vi "EXECUTE SWERVE DRIVE.vi"(0 "Swerve refs":cluster{"Driver":T1, "Steer":T1, "Encoder":T6}[](array[cluster]), 5 "HEADING":dbl, 7 "DRIVE MAX SPEED":dbl=0.7, 9 "STEER MAX speed":dbl=0.7) -> (4 "VELOCITIES":dbl[](array[numeric]), 6 "STEERING\nANGLES (deg)":dbl[](array[numeric]))   [LabVIEW 2023]
uses:
  <vilib>/Rock Robotics/WPI/MotorControl/WPI_MotorControlDeviceRef.ctl
  <vilib>/Rock Robotics/WPI/MotorControl/WPI_MotorControlType.ctl
  <vilib>/Rock Robotics/SystemInterfaces/DIO/FPGA_DIOPWMChannel.ctl
  <vilib>/Rock Robotics/WPI/PWM/WPI_PWMDeadband.ctl
  <vilib>/Rock Robotics/SystemInterfaces/DIO/FPGA_DIOChannel.ctl
  <vilib>/Rock Robotics/WPI/ThirdParty/Phoenix-LabVIEW/CANCoder/Controls/CTRE_Phoenix_CANcoder_DeviceRef.ctl
  <vilib>/Rock Robotics/WPI/ThirdParty/REV Robotics/REVLib/Typedef/Spark MAX Control Type.ctl
  Global odometry.vi
  Global INIT.vi
panel:
  out "error out":errorcluster
  in  "error in (no error)":errorcluster
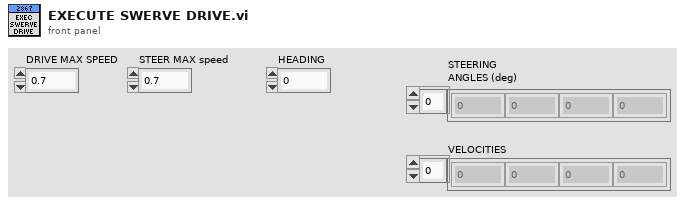
[diagram p1: front panel]
types:
  T1 = typedef "WPI_MotorControlDeviceRef.ctl" = cluster{"DeviceStatus":errorcluster, "Type":T2, "PWM":cluster{"PWM Channel":T3, "DeadBand":T4}, "CAN":cluster{"Device Number":u8, "SetOutput VI Ref":variant, "GetOutput VI Ref":variant, "Enable VI Ref":variant, "Disable VI Ref":variant, "Data":variant}, "Invert":bool, "DIO PWM":cluster{"PWM \"Enable\" Channel":T3, "DIOChannel":T5, "PWM Rate":dbl}}
  T2 = typedef "WPI_MotorControlType.ctl" = enum16{"PWM", "CAN", "DIO PWM"}
  T3 = typedef "FPGA_DIOPWMChannel.ctl" = enum8{"PWM 0", "PWM 1", "PWM 2", "PWM 3", "PWM 4", "PWM 5", "PWM 6", "PWM 7", "PWM 8", "PWM 9", "PWM MXP 0", "PWM MXP 1", "PWM MXP 2", "PWM MXP 3", "PWM MXP 4", "PWM MXP 5", "PWM MXP 6", "PWM MXP 7", "PWM MXP 8", "PWM MXP 9", "Invalid"}
  T4 = typedef "WPI_PWMDeadband.ctl" = cluster{"Name":string, "maxPositivePwm":i32, "minPositivePwm":i32, "centerPwm":i32, "maxNegativePwm":i32, "minNegativePwm":i32, "angularRange":u16}
  T5 = typedef "FPGA_DIOChannel.ctl" = enum8{"DIO 0", "DIO 1", "DIO 2", "DIO 3", "DIO 4", "DIO 5", "DIO 6", "DIO 7", "DIO 8", "DIO 9", "DIO MXP 0", "DIO MXP 1", "DIO MXP 2", "DIO MXP 3", "DIO MXP 4", "DIO MXP 5", "DIO MXP 6", "DIO MXP 7", "DIO MXP 8", "DIO MXP 9", "DIO MXP 10", "DIO MXP 11", "DIO MXP 12", "DIO MXP 13", "DIO MXP 14", "DIO MXP 15", "SPI Port CS1", "SPI Port CS2", "SPI Port CS3", "SPI Port MISO", "SPI Port MOSI", "Invalid"}
  T6 = typedef "CTRE_Phoenix_CANcoder_DeviceRef.ctl" = cluster{"DeviceStatus":errorcluster, "Device Number":u8, "Handle":u64, "UsageFrame":u32, "Library Path":path}
  T7 = typedef "ctrl pivot select.ctl" = enum16{"geometric center", "CG", "FL", "FR", "RR", "RL", "other"}
  T8 = typedef "ctrl XY coord.ctl" = cluster{"X":dbl, "Y":dbl}
  T9 = typedef "ctrl driver input.ctl" = cluster{"Jx":dbl, "Jy":dbl, "Jr ":dbl, "R":dbl, "theta (deg)":dbl, "theta (rad)":dbl, "PARK":bool}
  T10 = typedef "ctrl DRIVING FRAME selector.ctl" = enum16{"ROBO-centric", "FLD-centric"}
  T11 = typedef "ctrl FRONT FACE selector.ctl" = enum16{"intake side", "shooter side"}
  T12 = typedef "WPI_DriverStationAllianceInfo.ctl" = enum16{"Red", "Blue", "Invalid"}
  T13 = typedef "ctrl swerve motor.ctl" = cluster{"description":string, "MOTOR SELECT":T14, "Installed?":bool, "CAN ID":u8, "refnum name":string, "Invert":bool, "Idle Mode":T15, "Current limiting":T16, "MOTOR PIDF coefficients":T17, "gear ratio":dbl}
  T14 = typedef "ctrl MOTOR SELECT.ctl" = i16
  T15 = typedef "Spark MAX Idle Mode.ctl" = enum16{"Coast", "Brake"}
  T16 = typedef "ctrl Spark MAX current limiting.ctl" = cluster{"Linearized":bool, "Free Speed (A)":dbl, "Primay (A)":dbl, "Limit RPM (0)":u32}
  T17 = typedef "ctrl motor PIDF coefficients.ctl" = cluster{"PIDF":cluster{"P Gain":dbl, "I Gain":dbl, "D Gain":dbl, "F Gain":dbl, "I Zone":dbl, "Min Output":dbl, "Max Output":dbl}, "Smart Motion":T18}
  T18 = typedef "Spark MAX Smart Motion Parameters.ctl" = cluster{"Max Velocity":dbl, "Max Acceleration":dbl, "Minimum Velocity Output":dbl, "Allowed Closed Loop Error":dbl}
  T19 = typedef "ctrl swerve module.ctl" = cluster{"descr":string, "V":dbl, "POS":dbl, "target":dbl, "ABS":dbl, "from pivot to module":cluster{"R":dbl, "theta (deg)":dbl, "theta spin (deg)":dbl, "theta park (deg)":dbl}, "coord wrt geom CTR":cluster{"X":dbl, "Y":dbl}, "corner wt (lbm)":dbl}
  T20 = typedef "Spark MAX Control Type.ctl" = enum16{"Percent VBus", "Voltage", "Velocity", "Position", "Smart Motion", "Current", "Smart Velocity"}
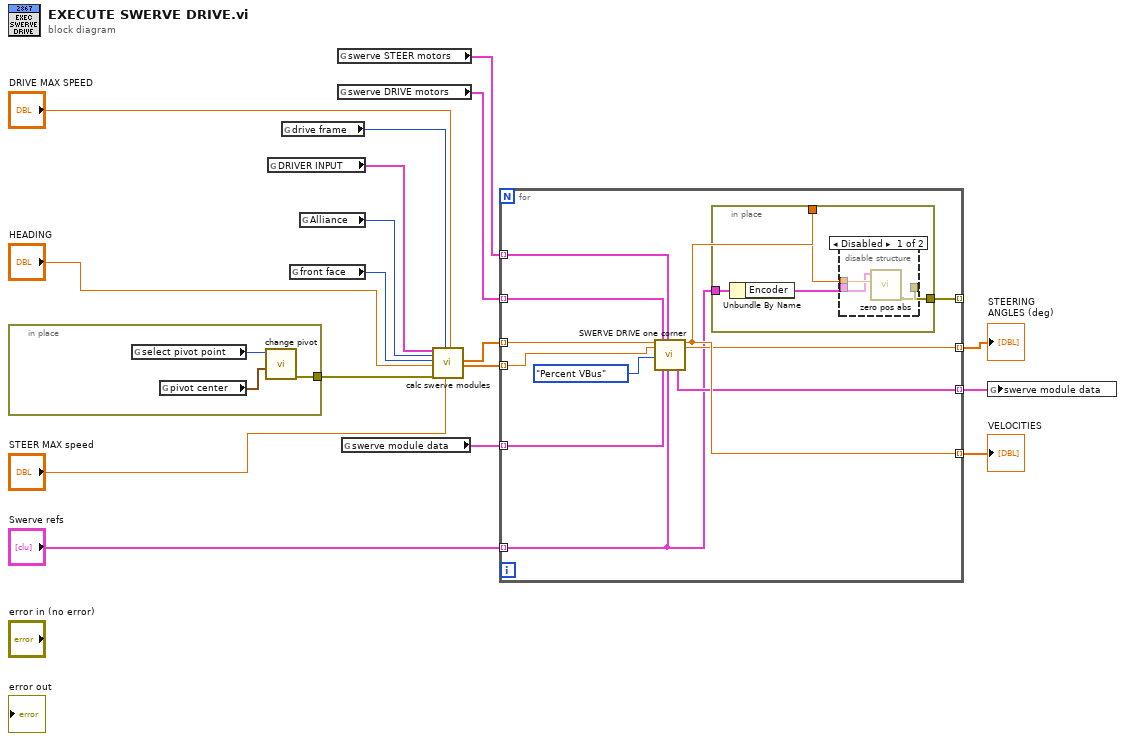
[diagram p0: block diagram]
diagram:
  n1 = in-place {
    in-place-border: [w18] -> w3
    n2 = global read "Global odometry.vi" "select pivot point"() -> (w20:T7)
    n3 = global read "Global odometry.vi" "pivot center"() -> (w19:T8)
    n4 = call "change pivot.vi"("new pivot center"=w19, "select pivot point"=w20) -> ("error out"=w18:errorcluster)  [unwired: 9 in]
  }
  n5 = global read "Global odometry.vi" "DRIVER INPUT"() -> (w4:T9)
  n6 = global read "Global odometry.vi" "drive frame"() -> (w7:T10)
  n7 = global read "Global odometry.vi" "front face"() -> (w5:T11)
  n8 = global read "Global odometry.vi" "Alliance"() -> (w6:T12)
  n9 = global read "Global INIT.vi" "swerve STEER motors"() -> (w2:T13[])
  n10 = global read "Global INIT.vi" "swerve DRIVE motors"() -> (w1:T13[])
  n11 = global read "Global odometry.vi" "swerve module data"() -> (w11:T19[])
  n12 = call "calc swerve modules.vi"("DRIVER INPUT"=w4, "Alliance"=w6, "front face"=w5, "HDG (deg)"="HEADING", "error in (no error)"=w3, "drive frame"=w7, "MAX spin (rev/s)"="STEER MAX speed", "Vmax"="DRIVE MAX SPEED") -> ("speed norm"=w9:dbl[], "angle"=w8:dbl[])  [unwired: 9 in, 1 out]
  n13 = for {
    tunnel: "Swerve refs" -> [w21] mode=indexing
    tunnel: w11 -> [w26] mode=indexing
    tunnel: [w29] -> w10 mode=indexing
    tunnel: w9 -> [w25] mode=indexing
    tunnel: w8 -> [w24] mode=indexing
    tunnel: [w30] -> w13 mode=indexing
    tunnel: [w31] -> w14 mode=indexing
    tunnel: w2 -> [w27] mode=indexing
    tunnel: w1 -> [w28] mode=indexing
    tunnel: [w22] -> _ mode=indexing
    n14 = call "SWERVE DRIVE one corner.vi"("velocity in"=w25, "steer angle in\n(deg)"=w24, "Control Mode"=Spark_MAX_Control_Type."Percent VBus", "drive\nmotor"=w28, "swerve module in"=w26, "steering\nmotor"=w27, "DeviceRefs"=w21) -> ("swerve module out"=w29:T19, "velocity out"=w31:dbl, "steer angle out\n(deg)"=w30:dbl)  [unwired: 9 in, 1 out]
    n15 = in-place {
      in-place-border: w31 -> [w35]
      in-place-border: w21 -> [w34]
      in-place-border: [w32] -> w22
      n16 = Unbundle By Name(w34) -> ("Encoder"=w33:T6)
      n17 = disable-structure shown="Disabled" {
        disable-tunnel: w35 -> [w38 _]
        disable-tunnel: w33 -> [w37 _]
        disable-tunnel: [w36 _] -> w32
        frame Disabled {
          n18 = call "zero pos abs.vi"("velocity"=w38, "Encoder"=w37) -> ("error out"=w36:errorcluster)  [unwired: 9 in]
        }
        frame Enabled {
        }
      }
    }
  }
  "VELOCITIES" <- w14
  "STEERING\nANGLES (deg)" <- w13
  n19 = global write "Global odometry.vi" "swerve module data"(w10) -> ()
